vi "GetZ (SubVI).vi"(8 "calibration":sgl, 10 "Data":sgl[][](array[numeric]), 11 "Array":i32[](array[numeric])) -> (0 "z":sgl, 2 "appended array":sgl[](array[numeric]), 4 "y":i32, 6 "x":i32)   [LabVIEW 2014]
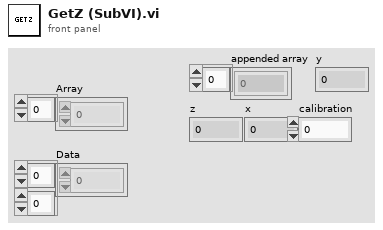
[diagram p1: front panel]
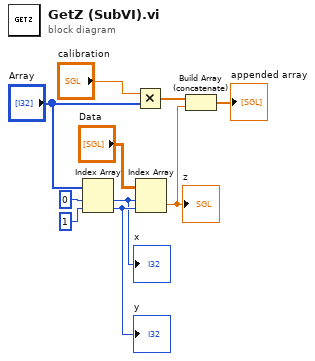
[diagram p0: block diagram]
diagram:
  n1 = Index Array(array="Array", index #1=0 ("index"), index #2=1 ("index")) -> (element #1=w9:i32, element #2=w10:i32)
  "x" <- w9
  "y" <- w10
  n2 = Multiply(x="calibration", y="Array") -> (x*y=w2:sgl[])
  n3 = Index Array(array="Data", index (row)=w9, index (col)=w10) -> (element=w4:sgl)
  "z" <- w4
  n4 = Build Array (concatenate)(w2, w4) -> (→"appended array":sgl[])
